vi "Message Maker.vi"(8 "error in (no error)":errorcluster, 10 "Actors Tree ref":refnum<vi>) -> (0 "error out":errorcluster, 1 "Active Project":i32, 2 "Projects":string[](array[string]), 3 "Message Maker out":refnum<class "Message Maker.lvclass">)   [LabVIEW 2023, in "Message Maker.lvclass"]
doc: "Constructs the message maker object. This will empty the tree and initialize the selected project\n\nAuthor: Derek Trepanier\nCopyright: MGI 2015"
uses:
  Message Maker.lvclass
  Message Maker.lvclass/Message Maker.ctl
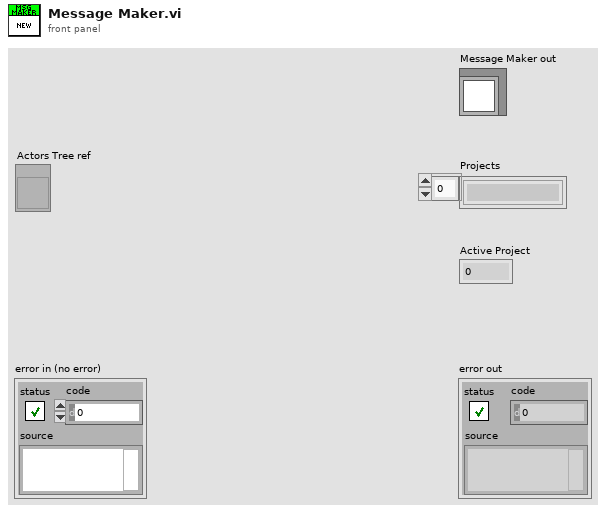
[diagram p1: front panel]
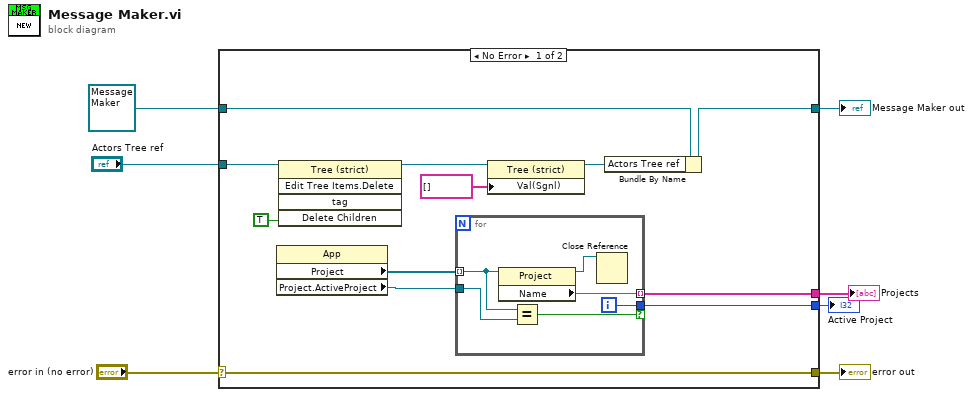
[diagram p0: block diagram]
diagram:
  n1 = case shown="No Error" "error in (no error)" {
    selector: "error in (no error)" -> [w19 w27]
    tunnel: [w19 w27] -> w6
    tunnel: [w15 w26] -> w4
    tunnel: refnum<class "Message Maker.lvclass"> refnum ("Message Maker in") -> [w18 w26]
    tunnel: [w16 _] -> w3
    tunnel: "Actors Tree ref" -> [w14 _]
    tunnel: [w9 _] -> w2
    frame No Error {
      n2 = property class="App"() -> ("Project"=w17:refnum<vi>[], "Project.ActiveProject"=w10:refnum<vi>)  [unwired: 2 in, 2 out]
      n3 = invoke class="Tree (strict)" method="Edit Tree Items.Delete"(reference=w14, "Delete Children"=TRUE ("Delete Children?")) -> (reference out=w13:refnum<vi>)  [unwired: 3 in, 4 out]
      n4 = for {
        tunnel: w17 -> [w24] mode=indexing
        tunnel: [w22] -> w16 mode=indexing
        tunnel: w10 -> [w23]
        tunnel: [w20] -> w9 if=w21
        i -> [w20]
        n5 = property class="Project"(reference=w24) -> (reference out=w25:refnum<vi>, "Name"=w22:string)  [unwired: 1 in, 1 out]
        n6 = Equal?(x=w24, y=w23) -> (x = y?=w21:bool)
        n7 = Close Reference(reference=w25) -> ()  [unwired: 1 in, 1 out]
      }
      n8 = property class="Tree (strict)"(reference=w13, "Val(Sgnl)"=string[] [] ("Value (Signaling)")) -> (reference out=w11:refnum<vi>)  [unwired: 1 in, 1 out]
      n9 = Bundle By Name(cluster=w18, "Actors Tree ref"=w11) -> (w15:refnum<class "Message Maker.lvclass">)
    }
    frame Error {
    }
  }
  "error out" <- w6
  "Message Maker out" <- w4
  "Projects" <- w3
  "Active Project" <- w2
